vi "kalman pv predict step fixed gain.vi"(11 "Kalman PV state":T1) -> (3 "Kalman PV state out":T1)   [LabVIEW 2010]
uses:
  kalman pv state.ctl
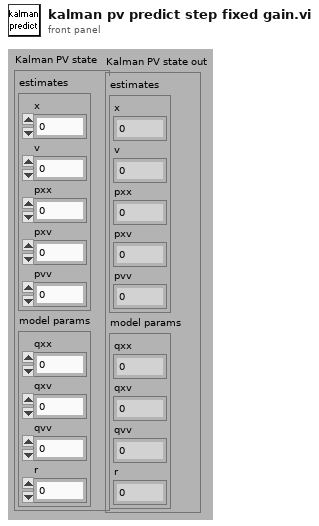
[diagram p1: front panel]
types:
  T1 = typedef "kalman pv state.ctl" = cluster{"estimates":cluster{"x":fxp<+/-,18,16>, "v":fxp<+/-,18,16>, "pxx":u16, "pxv":u16, "pvv":u16}, "model params":cluster{"qxx":u16, "qxv":u16, "qvv":u16, "r":u16}}
  T2 = cluster{"x":fxp<+/-,18,16>, "v":fxp<+/-,18,16>, "pxx":u16, "pxv":u16, "pvv":u16}
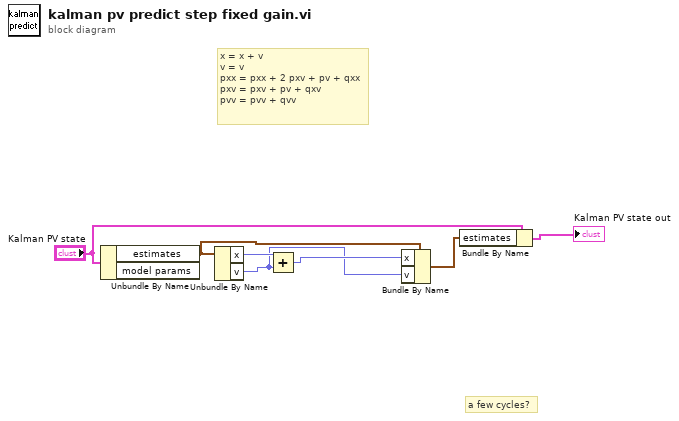
[diagram p0: block diagram]
diagram:
  # "a few cycles?"
  # "x = x + v\nv = v\npxx = pxx + 2 pxv + pv + qxx\npxv = pxv + pv + qxv\npvv = pvv + qvv"
  n1 = Unbundle By Name("Kalman PV state") -> ("estimates"=w6:T2)  [unwired: 1 out]
  n2 = Unbundle By Name(w6) -> ("x"=w7:fxp<+/-,18,16>, "v"=w4:fxp<+/-,18,16>)
  n3 = Add(x=w7, y=w4) -> (x+y=w5:fxp<+/-,18,16>)
  n4 = Bundle By Name(cluster=w6, "x"=w5, "v"=w4) -> (w3:T2)
  n5 = Bundle By Name(cluster="Kalman PV state", "estimates"=w3) -> (→"Kalman PV state out":T1)
